vi "mxwScript_Cmnd2Str_connectWire.vi"(8 "error in (no error)":errorcluster, 11 "data":variant) -> (0 "error out":errorcluster, 3 "outputString":string)   [LabVIEW 2017]
uses:
  codeGenAPISupport.llb/cgAPI_mxwScript_Wire_WireConnection.ctl
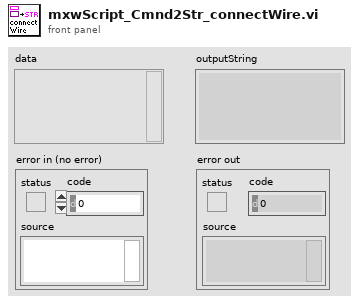
[diagram p1: front panel]
types:
  T1 = typedef "cgAPI_mxwScript_Wire_WireConnection.ctl" = cluster{"source":string, "source index":i32, "sink":string, "sink index":i32}
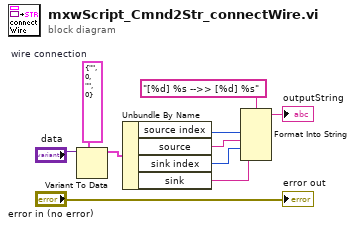
[diagram p0: block diagram]
diagram:
  w7 = T1 {"source"="", "source index"=0, "sink"="", "sink index"=0}  # wire connection
  n1 = Variant To Data(type=w7, Variant="data") -> (data=w9:T1)  [unwired: 1 in, 1 out]
  n2 = Unbundle By Name(w9) -> ("source index"=w5:i32, "source"=w3:string, "sink index"=w2:i32, "sink"=w4:string)
  n3 = Format Into String(format string="[%d] %s -->> [%d] %s", w5, w3, w2, w4) -> (resulting string=→"outputString":string)  [unwired: 2 in, 1 out]
  "error out" <- "error in (no error)"
